vi "Perform Action.vi"(7 "Instrument":refnum<class "Instrument.lvclass">, 8 "error in":errorcluster, 10 "Input":variant, 11 "object in":refnum<class "Perform Action Remote on Const Channel with 2DBL Strategy.lvclass">) -> (0 "error out":errorcluster, 2 "Output":variant, 3 "object out":refnum<class "Perform Action Remote on Const Channel with 2DBL Strategy.lvclass">)   [LabVIEW 2024, in "HAL.lvlib" / "Perform Action Remote on Const Channel with 2DBL Strategy.lvclass"]
uses:
  Perform Action Remote on Const Channel with 2DBL Strategy.lvclass
  Instrument/Instrument.lvclass
  PA on Const Channel Strategy/Perform Action on Const Channel Strategy.lvclass/Perform Action on Const Channel Strategy.ctl
  PA on Const Channel Strategy/Perform Action on Const Channel Strategy.lvclass
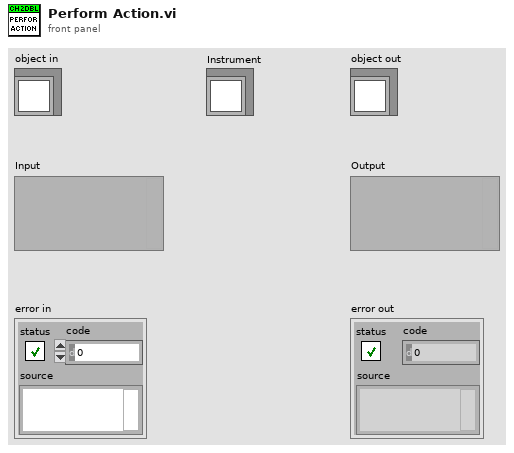
[diagram p1: front panel]
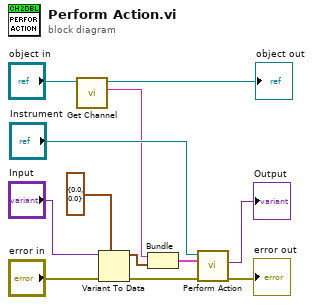
[diagram p0: block diagram]
diagram:
  n1 = call "Get Channel.vi"("Perform Action on Const Channel Strategy in"="object in") -> ("Channel"=w1:string, "Perform Action on Const Channel Strategy out"=→"object out":refnum<class "Perform Action Remote on Const Channel with 2DBL Strategy.lvclass">)  [unwired: 9 in]
  n2 = Variant To Data(error in="error in", type=cluster{dbl, dbl} {0.0, 0.0}, Variant="Input") -> (data=w6:cluster{dbl, dbl}, error out=w10:errorcluster)
  n3 = Bundle("Channel"=w1, w6) -> (w5:cluster{"Channel":string, cluster{dbl, dbl}})  [unwired: 1 in]
  n4 = call "Perform Action.vi"("Error In"=w10, "Input"=w5, "reference in"="Instrument") -> ("Error Out"=→"error out":errorcluster, "Output"=→"Output":variant)  [unwired: 6 in, 1 out]
